vi "Check File Exits and Create.vi"(8 "error in":errorcluster, 11 "Path In":path) -> (0 "error out":errorcluster, 1 "file exists?":bool, 2 "refnum out":refnum<file>, 3 "Path Out":path)   [LabVIEW 2019]
panel:
  # "Voltage Calibration-1.txt"
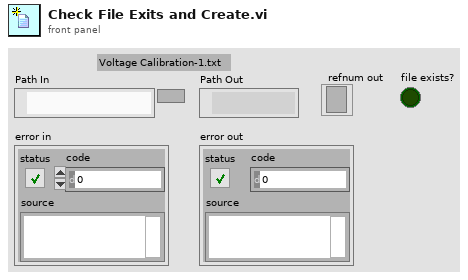
[diagram p1: front panel]
types:
  T1 = enum16{"open", "replace", "create", "open or create", "replace or create", "replace or create with confirmation"}
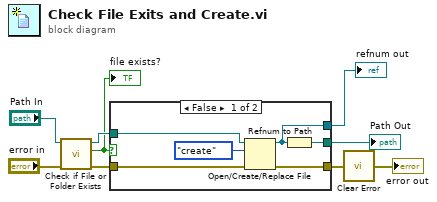
[diagram p0: block diagram]
diagram:
  n1 = call <vilib>:"Check if File or Folder Exists.vi"("error in (no error)"="error in", "path"="Path In") -> ("error out"=w7:errorcluster, "file or folder exists?"=w5:bool, "dup path"=w6:path)  [unwired: 7 in]
  "file exists?" <- w5
  n2 = case shown="False" w5 {
    tunnel: w6 -> [w15 w17]
    tunnel: w7 -> [w14 w16]
    tunnel: [w12 w16] -> w9
    tunnel: [w11 w17] -> w8
    tunnel: [w10 _] -> w2
    frame False {
      n3 = Open/Create/Replace File(file path (use dialog)=w15, error in=w14, operation (0:open)=T1."create") -> (refnum out=w10:refnum<file>, error out=w12:errorcluster)  [unwired: 3 in, 1 out]
      n4 = Refnum to Path(1:w10) -> (0:w11:path)
    }
    frame True {
    }
  }
  "Path Out" <- w8
  "refnum out" <- w2
  n5 = call "Clear Error.vi"("error in"=w9) -> ("error out"=→"error out":errorcluster)
